vi "Data Source Select.vi"(11 "Data Path":path) -> (2 "Add Data Source":string[](array[string]), 3 "OK？":bool)   [LabVIEW 2020]
uses:
  <vilib>/Utility/file.llb/Read Delimited Spreadsheet (string).vi
panel:
  in  "Export":bool
  in  "Import":bool
  in  "Selected Data Source":i32(listbox)
  out "Title":bool
  in  "OK":bool
  in  "Cancel":bool
  in  "Data Source List":i32(listbox)
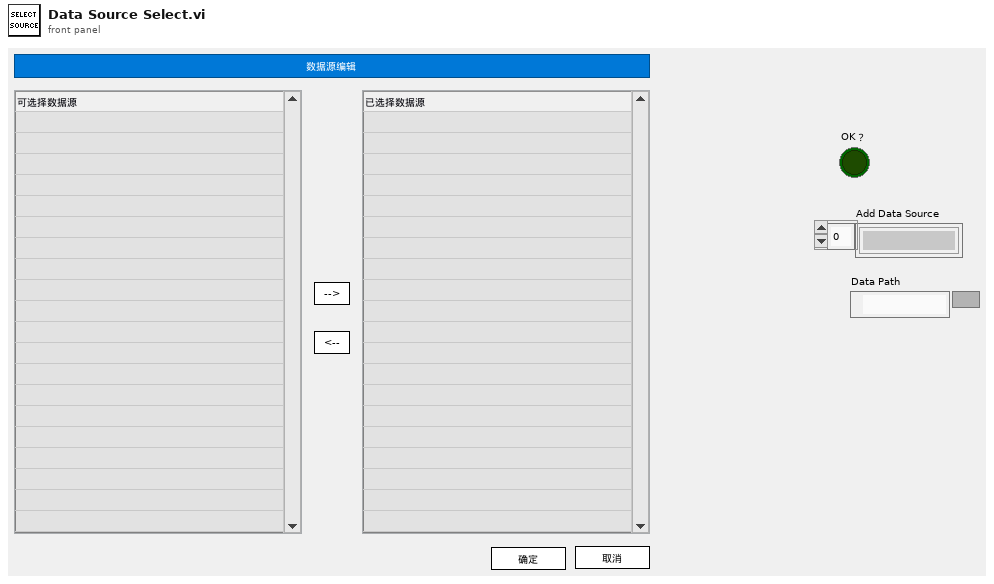
[diagram p1: front panel]
types:
  T1 = cluster{"Add Data Source":string[], "Data Source List":string[], "Timeout":i32, "OK？":bool, "Exit":bool, "Data Source List":i32, "Selected Data Source":i32}
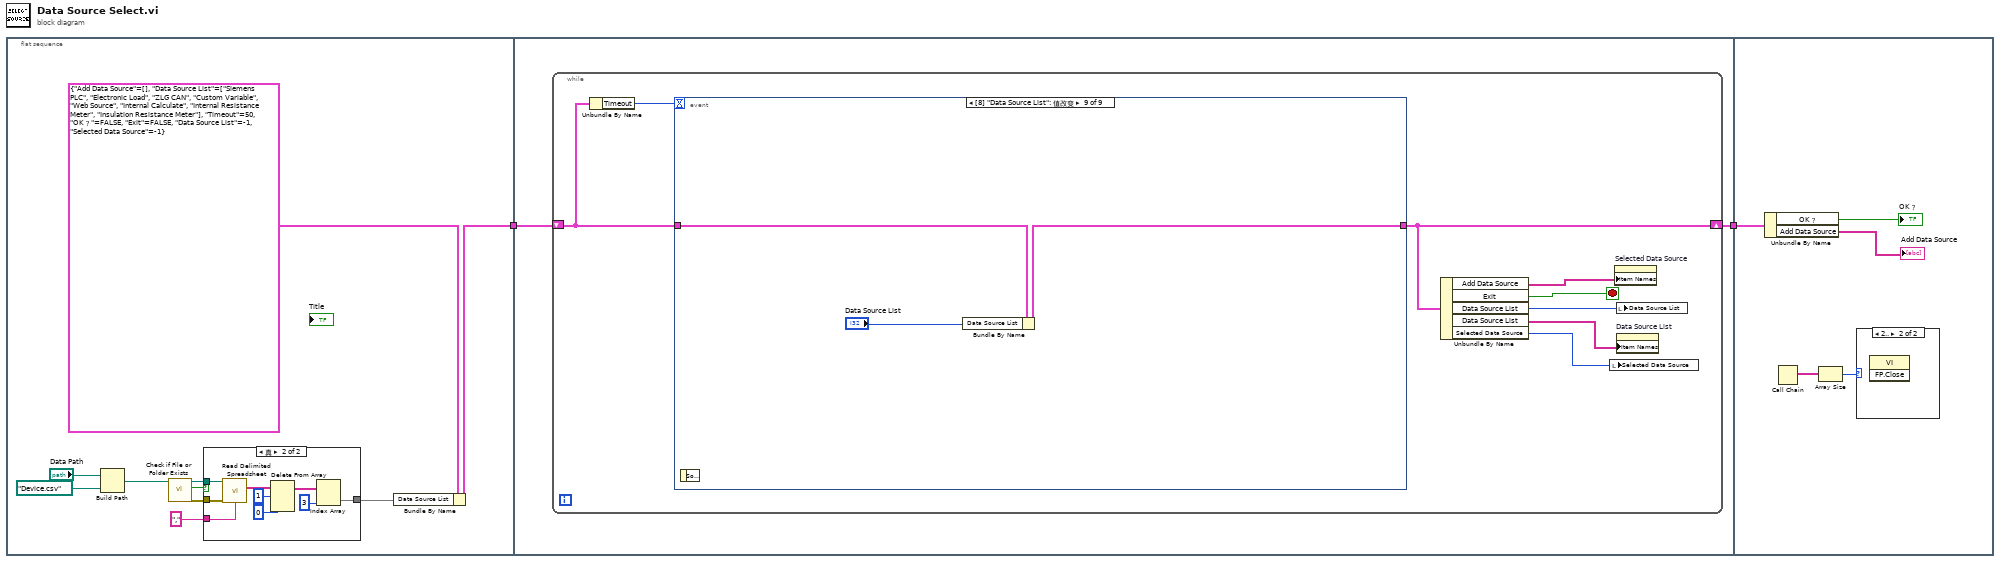
[diagram p0: block diagram]
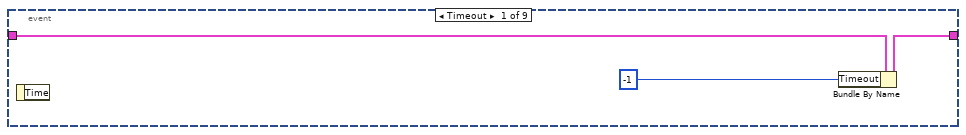
[diagram p3: hidden frame]
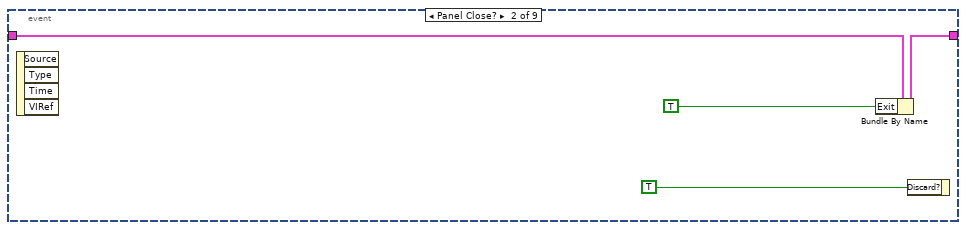
[diagram p4: hidden frame]
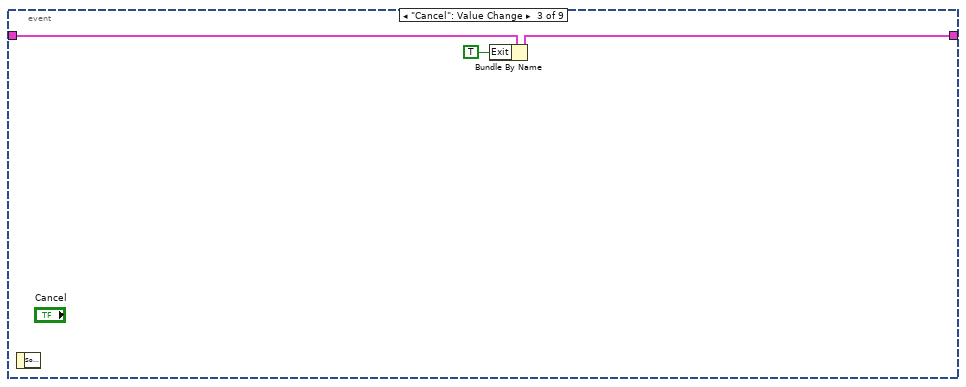
[diagram p5: hidden frame]
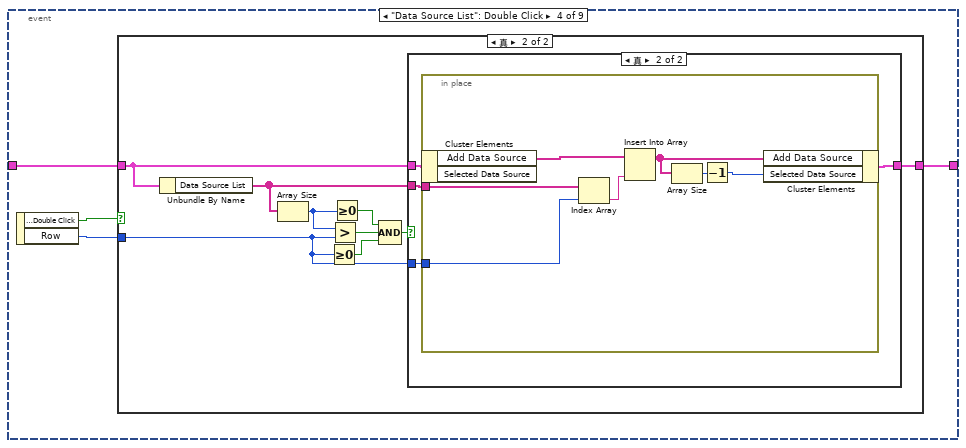
[diagram p6: hidden frame]
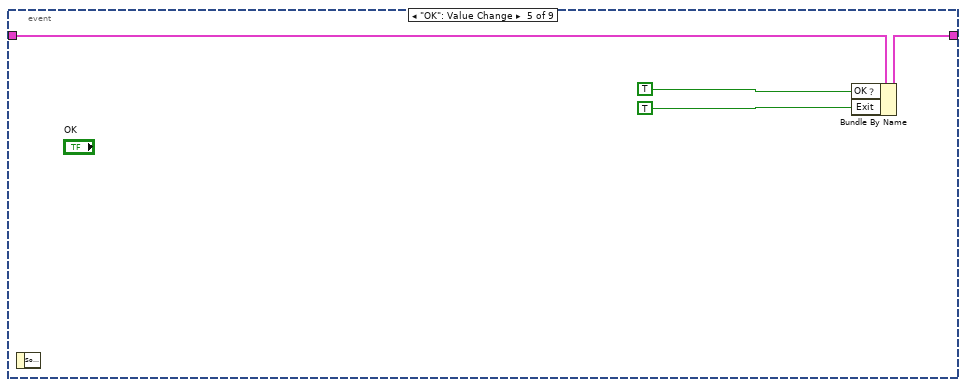
[diagram p9: hidden frame]
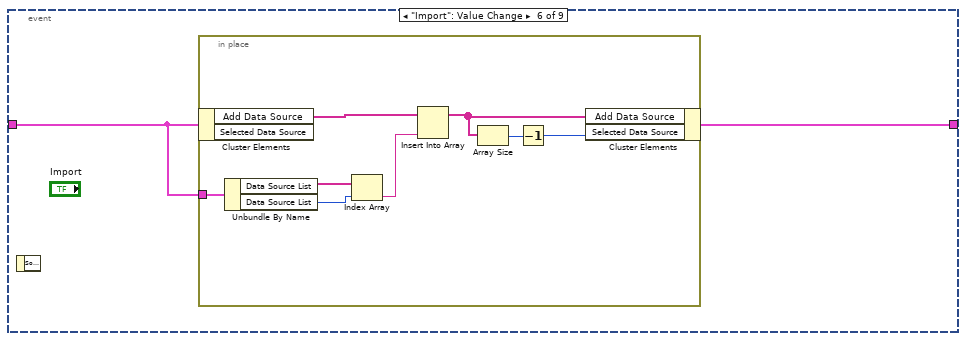
[diagram p10: hidden frame]
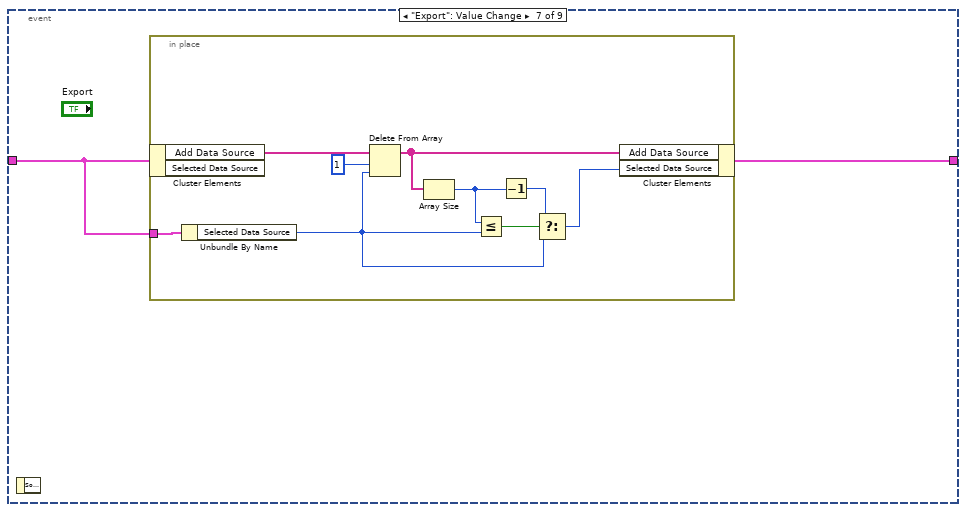
[diagram p11: hidden frame]
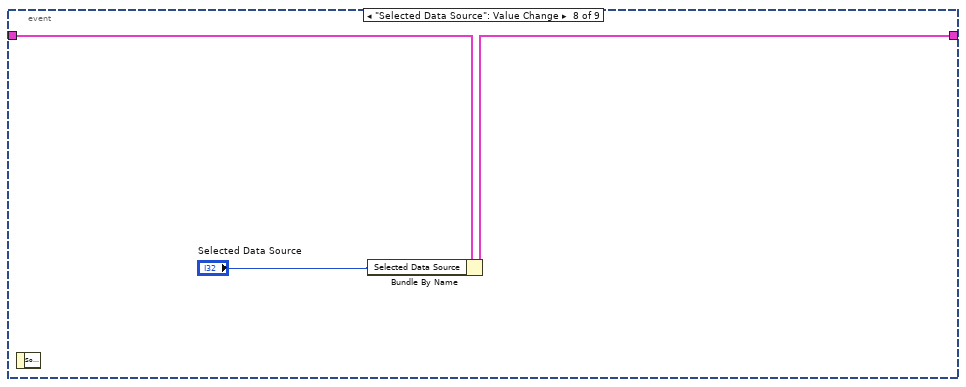
[diagram p12: hidden frame]
diagram:
  n1 = flat-sequence {
    tunnel: [w7] -> w2
    tunnel: w2 -> [w23]
    tunnel: [w22] -> w1
    tunnel: w1 -> [w101]
    frame #0 {
      n2 = Build Path(base path="Data Path", name or relative path=path "Device.csv" ("名称或相对路径")) -> (appended path=w4:path)
      n3 = call <vilib>:"Check if File or Folder Exists.vi"("path"=w4) -> ("error out"=w9:errorcluster, "file or folder exists?"=w11:bool, "dup path"=w10:path)  [unwired: 8 in]
      n4 = case shown="真" w11 {
        tunnel: w10 -> [_ w21]
        tunnel: w9 -> [_ w19]
        tunnel: "," ("delimiter (\\t)") -> [_ w20]
        tunnel: [_ w13] -> w6
        frame False {
        }
        frame True {
          n5 = call-poly <vilib>:"Read Delimited Spreadsheet.vi"("file path (dialog if empty)"=w21, "error in (no error)"=w19, "delimiter (\\t)"=w20) -> ("all rows"=w18:string[][])  [unwired: 7 in, 5 out]
          n6 = Delete From Array(array=w18, length=1 ("长度"), index (row)=0 ("索引 (行)")) -> (array with subset deleted=w17:string[][])  [unwired: 1 in, 1 out]
          n7 = Index Array(array=w17, index (col)=3 ("禁用的索引 (列)")) -> (element=w13:string[])  [unwired: 1 in]
        }
      }
      n8 = Bundle By Name(cluster=T1 {"Add Data Source"=[], "Data Source List"=["Siemens PLC", "Electronic Load", "ZLG CAN", "Custom Variable", "Web Source", "Internal Calculate", "Internal Resistance Meter", "Insulation Resistance Meter"], "Timeout"=50, "OK？"=FALSE, "Exit"=FALSE, "Data Source List"=-1, "Selected Data Source"=-1}, "Data Source List"=w6) -> (w7:T1)
    }
    frame #1 {
      n9 = while {
        shift-right: [w31] -> w22
        shift-left: w23 -> [w29]
        stop <- w27 stop-if-true
        n10 = Unbundle By Name(w29) -> ("Timeout"=w28:i32)
        n11 = event shown="[8] \"Data Source List\": 值改变" {
          selector: _ -> [_ _ _ _ _ _ _ _ _]
          dyn-events: _ -> [_ _ _ _ _ _ _ _ _]
          timeout: w28 -> [_ _ _ _ _ _ _ _ _]
          tunnel: w29 -> [w34 w37 w41 w45 w71 w72 w82 w95 w98]
          tunnel: [w33 w36 w40 w44 w70 w73 w83 w94 w97] -> w31
          event Timeout {
            n12 = event-data() -> ()  [unwired: 1 in, 1 out]
            n13 = Bundle By Name(cluster=w34, "Timeout"=-1) -> (w33:T1)
          }
          event Panel Close? {
            n14 = event-data() -> ()  [unwired: 1 in, 4 out]
            n15 = Bundle By Name(cluster=w37, "Exit"=TRUE) -> (w36:T1)
            n16 = event-data("Discard?"=TRUE ("放弃？")) -> ()  [unwired: 1 in, 1 out]
          }
          event "Cancel": Value Change {
            n17 = event-data() -> ()  [unwired: 1 in, 1 out]
            n18 = Bundle By Name(cluster=w41, "Exit"=TRUE) -> (w40:T1)
          }
          event "Data Source List": Double Click {
            n19 = event-data() -> ("Mods.Double Click"=w43:bool, "Row"=w42:i32)  [unwired: 1 in]
            n20 = case shown="真" w43 {
              tunnel: w45 -> [w46 w54]
              tunnel: [w46 w55] -> w44
              tunnel: w42 -> [_ w47]
              frame False {
              }
              frame True {
                n21 = Unbundle By Name(w54) -> ("Data Source List"=w48:string[])
                n22 = Array Size(array=w48) -> (size(s)=w53:i32)
                n23 = Greater Or Equal To 0?(x=w47) -> (x >= 0?=w50:bool)
                n24 = Greater?(x=w53, y=w47) -> (0:w51:bool)
                n25 = Greater Or Equal To 0?(x=w53) -> (x >= 0?=w52:bool)
                n26 = Compound Arithmetic op=AND ("复合运算")(w52, w51, w50) -> (w49:bool)
                n27 = case shown="真" w49 {
                  tunnel: [w56 w60] -> w55
                  tunnel: w54 -> [w56 w59]
                  tunnel: w48 -> [_ w58]
                  tunnel: w47 -> [_ w57]
                  frame False {
                  }
                  frame True {
                    n28 = in-place {
                      in-place-border: w58 -> [w67]
                      in-place-border: w57 -> [w66]
                      n29 = in-place-cluster #1(w59) -> ("Add Data Source"=w65:string[])  [unwired: 1 out]
                      n30 = Index Array(array=w67, index=w66) -> (element=w64:string)
                      n31 = Insert Into Array(array=w65, new element=w64) -> (w63:string[])  [unwired: 1 in]
                      n32 = Array Size(array=w63) -> (size(s)=w62:i32)
                      n33 = Decrement(x=w62) -> (x-1=w61:i32)
                      n34 = in-place-cluster #1("Add Data Source"=w63, "Selected Data Source"=w61) -> (w60:T1)
                    }
                  }
                }
              }
            }
          }
          event "OK": Value Change {
            n35 = event-data() -> ()  [unwired: 1 in, 1 out]
            n36 = Bundle By Name(cluster=w71, "OK？"=TRUE, "Exit"=TRUE) -> (w70:T1)
          }
          event "Import": Value Change {
            n37 = event-data() -> ()  [unwired: 1 in, 1 out]
            n38 = in-place {
              in-place-border: w72 -> [w78]
              n39 = in-place-cluster #2(w72) -> ("Add Data Source"=w81:string[])  [unwired: 1 out]
              n40 = Unbundle By Name(w78) -> ("Data Source List"=w79:string[], "Data Source List"=w80:i32)
              n41 = Index Array(array=w79, index=w80) -> (element=w77:string)
              n42 = Insert Into Array(array=w81, new element=w77) -> (w76:string[])  [unwired: 1 in]
              n43 = Array Size(array=w76) -> (size(s)=w75:i32)
              n44 = Decrement(x=w75) -> (x-1=w74:i32)
              n45 = in-place-cluster #2("Add Data Source"=w76, "Selected Data Source"=w74) -> (w73:T1)
            }
          }
          event "Export": Value Change {
            n46 = event-data() -> ()  [unwired: 1 in, 1 out]
            n47 = in-place {
              in-place-border: w82 -> [w90]
              n48 = in-place-cluster #3(w82) -> ("Add Data Source"=w92:string[])  [unwired: 1 out]
              n49 = Unbundle By Name(w90) -> ("Selected Data Source"=w87:i32)
              n50 = Delete From Array(array=w92, length=1 ("长度"), index=w87) -> (array with subset deleted=w89:string[])  [unwired: 1 out]
              n51 = Array Size(array=w89) -> (size(s)=w86:i32)
              n52 = Less Or Equal?(x=w86, y=w87) -> (x <= y?=w88:bool)
              n53 = Decrement(x=w86) -> (x-1=w84:i32)
              n54 = Select(t=w84, s=w88, f=w87) -> (s? t:f=w85:i32)
              n55 = in-place-cluster #3("Add Data Source"=w89, "Selected Data Source"=w85) -> (w83:T1)
            }
          }
          event "Selected Data Source": Value Change {
            n56 = event-data() -> ()  [unwired: 1 in, 1 out]
            n57 = Bundle By Name(cluster=w95, "Selected Data Source"="Selected Data Source") -> (w94:T1)
          }
          event "Data Source List": Value Change {
            n58 = event-data() -> ()  [unwired: 1 in, 1 out]
            n59 = Bundle By Name(cluster=w98, "Data Source List"="Data Source List") -> (w97:T1)
          }
        }
        n60 = Unbundle By Name(w31) -> ("Add Data Source"=w30:string[], "Exit"=w27:bool, "Data Source List"=w26:i32, "Data Source List"=w25:string[], "Selected Data Source"=w24:i32)
        n61 = local write "Selected Data Source"(w24) -> ()
        n62 = property on="Selected Data Source" class="LstBox (严格)"("Item Names"=w30) -> ()  [unwired: 2 in, 2 out]
        n63 = local write "Data Source List"(w26) -> ()
        n64 = property on="Data Source List" class="LstBox (严格)"("Item Names"=w25) -> ()  [unwired: 2 in, 2 out]
      }
    }
    frame #2 {
      n65 = Unbundle By Name(w101) -> ("OK？"=→"OK？":bool, "Add Data Source"=→"Add Data Source":string[])
      n66 = Call Chain() -> (call chain=w103:string[])
      n67 = Array Size(array=w103) -> (size(s)=w102:i32)
      n68 = case shown="2.." w102 {
        frame 0, Default {
        }
        frame 2.. {
          n69 = invoke class="VI" method="FP.Close"() -> ()  [unwired: 3 in, 3 out]
        }
      }
    }
  }
